vi "getVolume.vi"(8 "error in (no error)":errorcluster, 11 "Radio in":refnum<class "Radio.lvclass">) -> (0 "error out":errorcluster, 2 "volume":i32, 3 "Radio out":refnum<class "Radio.lvclass">)   [LabVIEW 2017, in "Radio.lvclass"]
uses:
  Radio.lvclass
  Device Class/Device.lvclass
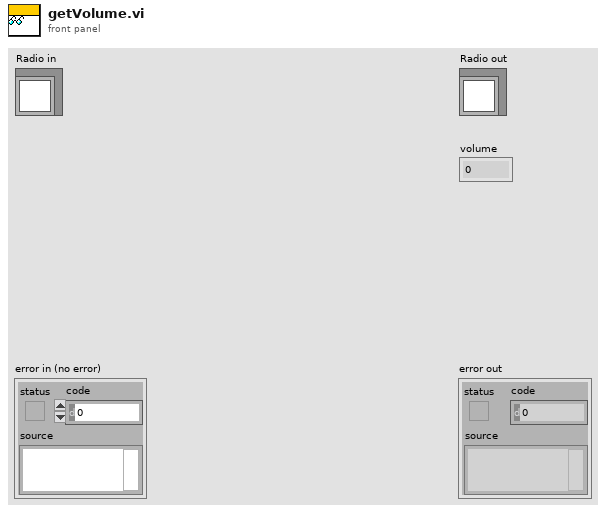
[diagram p1: front panel]
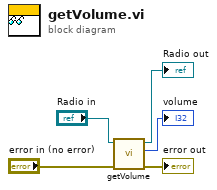
[diagram p0: block diagram]
diagram:
  n1 = call-parent "getVolume.vi"("error in (no error)"="error in (no error)", "Device in"="Radio in") -> ("error out"=→"error out":errorcluster, "volume"=→"volume":i32, "Device out"=→"Radio out":refnum<class "Radio.lvclass">)  [unwired: 7 in]
